vi "@create.vi"(4 "CodePage (<do not specify>)":i32(ring)=-1 items=["<do not specify>"=-1, "<use OEM Code Page>"=0, "IBM037 - IBM EBCDIC US-Canada"=37, "IBM437 - OEM United States"=437, "IBM500 - IBM EBCDIC International"=500, "ASMO-708 - Arabic (ASMO 708)"=708, "709 - Arabic (ASMO-449+, BCON V4)"=709, "710 - Arabic - Transparent Arabic"=710, "DOS-720 - Arabic (Transparent ASMO); Arabic (DOS)"=720, "ibm737 - OEM Greek (formerly 437G); Greek (DOS)"=737, "ibm775 - OEM Baltic; Baltic (DOS)"=775, "ibm850 - OEM Multilingual Latin 1; Western European (DOS)"=850, "ibm852 - OEM Latin 2; Central European (DOS)"=852, "IBM855 - OEM Cyrillic (primarily Russian)"=855, "ibm857 - OEM Turkish; Turkish (DOS)"=857, "IBM00858 - OEM Multilingual Latin 1 + Euro symbol"=858, "IBM860 - OEM Portuguese; Portuguese (DOS)"=860, "ibm861 - OEM Icelandic; Icelandic (DOS)"=861, "DOS-862 - OEM Hebrew; Hebrew (DOS)"=862, "IBM863 - OEM French Canadian; French Canadian (DOS)"=863, "IBM864 - OEM Arabic; Arabic (864)"=864, "IBM865 - OEM Nordic; Nordic (DOS)"=865, "cp866 - OEM Russian; Cyrillic (DOS)"=866, "ibm869 - OEM Modern Greek; Greek, Modern (DOS)"=869, "IBM870 - IBM EBCDIC Multilingual/ROECE (Latin 2); IBM EBCDIC Multilingual Latin 2"=870, "windows-874 - Thai (Windows)"=874, "cp875 - IBM EBCDIC Greek Modern"=875, "shift_jis - ANSI/OEM Japanese; Japanese (Shift-JIS)"=932, "gb2312 - ANSI/OEM Simplified Chinese (PRC, Singapore); Chinese Simplified (GB2312)"=936, "ks_c_5601-1987 - ANSI/OEM Korean (Unified Hangul Code)"=949, "big5 - ANSI/OEM Traditional Chinese (Taiwan; Hong Kong SAR, PRC); Chinese Traditional (Big5)"=950, "IBM1026 - IBM EBCDIC Turkish (Latin 5)"=1026, "IBM01047 - IBM EBCDIC Latin 1/Open System"=1047, "IBM01140 - IBM EBCDIC US-Canada (037 + Euro symbol); IBM EBCDIC (US-Canada-Euro)"=1140, "IBM01141 - IBM EBCDIC Germany (20273 + Euro symbol); IBM EBCDIC (Germany-Euro)"=1141, "IBM01142 - IBM EBCDIC Denmark-Norway (20277 + Euro symbol); IBM EBCDIC (Denmark-Norway-Euro)"=1142, "IBM01143 - IBM EBCDIC Finland-Sweden (20278 + Euro symbol); IBM EBCDIC (Finland-Sweden-Euro)"=1143, "IBM01144 - IBM EBCDIC Italy (20280 + Euro symbol); IBM EBCDIC (Italy-Euro)"=1144, "IBM01145 - IBM EBCDIC Latin America-Spain (20284 + Euro symbol); IBM EBCDIC (Spain-Euro)"=1145, "IBM01146 - IBM EBCDIC United Kingdom (20285 + Euro symbol); IBM EBCDIC (UK-Euro)"=1146, "IBM01147 - IBM EBCDIC France (20297 + Euro symbol); IBM EBCDIC (France-Euro)"=1147, "IBM01148 - IBM EBCDIC International (500 + Euro symbol); IBM EBCDIC (International-Euro)"=1148, "IBM01149 - IBM EBCDIC Icelandic (20871 + Euro symbol); IBM EBCDIC (Icelandic-Euro)"=1149, "utf-16 - Unicode UTF-16, little endian byte order (BMP of ISO 10646); available only to managed applications"=1200, "unicodeFFFE - Unicode UTF-16, big endian byte order; available only to managed applications"=1201, "windows-1250 - ANSI Central European; Central European (Windows)"=1250, "windows-1251 - ANSI Cyrillic; Cyrillic (Windows)"=1251, "windows-1252 - ANSI Latin 1; Western European (Windows)"=1252, "windows-1253 - ANSI Greek; Greek (Windows)"=1253, "windows-1254 - ANSI Turkish; Turkish (Windows)"=1254, "windows-1255 - ANSI Hebrew; Hebrew (Windows)"=1255, "windows-1256 - ANSI Arabic; Arabic (Windows)"=1256, "windows-1257 - ANSI Baltic; Baltic (Windows)"=1257, "windows-1258 - ANSI/OEM Vietnamese; Vietnamese (Windows)"=1258, "Johab - Korean (Johab)"=1361, "macintosh - MAC Roman; Western European (Mac)"=10000, "x-mac-japanese - Japanese (Mac)"=10001, "x-mac-chinesetrad - MAC Traditional Chinese (Big5); Chinese Traditional (Mac)"=10002, "x-mac-korean - Korean (Mac)"=10003, "x-mac-arabic - Arabic (Mac)"=10004, "x-mac-hebrew - Hebrew (Mac)"=10005, "x-mac-greek - Greek (Mac)"=10006, "x-mac-cyrillic - Cyrillic (Mac)"=10007, "x-mac-chinesesimp - MAC Simplified Chinese (GB 2312); Chinese Simplified (Mac)"=10008, "x-mac-romanian - Romanian (Mac)"=10010, "x-mac-ukrainian - Ukrainian (Mac)"=10017, "x-mac-thai - Thai (Mac)"=10021, "x-mac-ce - MAC Latin 2; Central European (Mac)"=10029, "x-mac-icelandic - Icelandic (Mac)"=10079, "x-mac-turkish - Turkish (Mac)"=10081, "x-mac-croatian - Croatian (Mac)"=10082, "utf-32 - Unicode UTF-32, little endian byte order; available only to managed applications"=12000, "utf-32BE - Unicode UTF-32, big endian byte order; available only to managed applications"=12001, "x-Chinese_CNS - CNS Taiwan; Chinese Traditional (CNS)"=20000, "x-cp20001 - TCA Taiwan"=20001, "x_Chinese-Eten - Eten Taiwan; Chinese Traditional (Eten)"=20002, "x-cp20003 - IBM5550 Taiwan"=20003, "x-cp20004 - TeleText Taiwan"=20004, "x-cp20005 - Wang Taiwan"=20005, "x-IA5 - IA5 (IRV International Alphabet No. 5, 7-bit); Western European (IA5)"=20105, "x-IA5-German - IA5 German (7-bit)"=20106, "x-IA5-Swedish - IA5 Swedish (7-bit)"=20107, "x-IA5-Norwegian - IA5 Norwegian (7-bit)"=20108, "us-ascii - US-ASCII (7-bit)"=20127, "x-cp20261 - T.61"=20261, "x-cp20269 - ISO 6937 Non-Spacing Accent"=20269, "IBM273 - IBM EBCDIC Germany"=20273, "IBM277 - IBM EBCDIC Denmark-Norway"=20277, "IBM278 - IBM EBCDIC Finland-Sweden"=20278, "IBM280 - IBM EBCDIC Italy"=20280, "IBM284 - IBM EBCDIC Latin America-Spain"=20284, "IBM285 - IBM EBCDIC United Kingdom"=20285, "IBM290 - IBM EBCDIC Japanese Katakana Extended"=20290, "IBM297 - IBM EBCDIC France"=20297, "IBM420 - IBM EBCDIC Arabic"=20420, "IBM423 - IBM EBCDIC Greek"=20423, "IBM424 - IBM EBCDIC Hebrew"=20424, "x-EBCDIC-KoreanExtended - IBM EBCDIC Korean Extended"=20833, "IBM-Thai - IBM EBCDIC Thai"=20838, "koi8-r - Russian (KOI8-R); Cyrillic (KOI8-R)"=20866, "IBM871 - IBM EBCDIC Icelandic"=20871, "IBM880 - IBM EBCDIC Cyrillic Russian"=20880, "IBM905 - IBM EBCDIC Turkish"=20905, "IBM00924 - IBM EBCDIC Latin 1/Open System (1047 + Euro symbol)"=20924, "EUC-JP - Japanese (JIS 0208-1990 and 0212-1990)"=20932, "x-cp20936 - Simplified Chinese (GB2312); Chinese Simplified (GB2312-80)"=20936, "x-cp20949 - Korean Wansung"=20949, "cp1025 - IBM EBCDIC Cyrillic Serbian-Bulgarian"=21025, "21027 - (deprecated)"=21027, "koi8-u - Ukrainian (KOI8-U); Cyrillic (KOI8-U)"=21866, "iso-8859-1 - ISO 8859-1 Latin 1; Western European (ISO)"=28591, "iso-8859-2 - ISO 8859-2 Central European; Central European (ISO)"=28592, "iso-8859-3 - ISO 8859-3 Latin 3"=28593, "iso-8859-4 - ISO 8859-4 Baltic"=28594, "iso-8859-5 - ISO 8859-5 Cyrillic"=28595, "iso-8859-6 - ISO 8859-6 Arabic"=28596, "iso-8859-7 - ISO 8859-7 Greek"=28597, "iso-8859-8 - ISO 8859-8 Hebrew; Hebrew (ISO-Visual)"=28598, "iso-8859-9 - ISO 8859-9 Turkish"=28599, "iso-8859-13 - ISO 8859-13 Estonian"=28603, "iso-8859-15 - ISO 8859-15 Latin 9"=28605, "x-Europa - Europa 3"=29001, "iso-8859-8-i - ISO 8859-8 Hebrew; Hebrew (ISO-Logical)"=38598, "iso-2022-jp - ISO 2022 Japanese with no halfwidth Katakana; Japanese (JIS)"=50220, "csISO2022JP - ISO 2022 Japanese with halfwidth Katakana; Japanese (JIS-Allow 1 byte Kana)"=50221, "iso-2022-jp - ISO 2022 Japanese JIS X 0201-1989; Japanese (JIS-Allow 1 byte Kana - SO/SI)"=50222, "iso-2022-kr - ISO 2022 Korean"=50225, "x-cp50227 - ISO 2022 Simplified Chinese; Chinese Simplified (ISO 2022)"=50227, "50229 - ISO 2022 Traditional Chinese"=50229, "50930 - EBCDIC Japanese (Katakana) Extended"=50930, "50931 - EBCDIC US-Canada and Japanese"=50931, "50933 - EBCDIC Korean Extended and Korean"=50933, "50935 - EBCDIC Simplified Chinese Extended and Simplified Chinese"=50935, "50936 - EBCDIC Simplified Chinese"=50936, "50937 - EBCDIC US-Canada and Traditional Chinese"=50937, "50939 - EBCDIC Japanese (Latin) Extended and Japanese"=50939, "euc-jp - EUC Japanese"=51932, "EUC-CN - EUC Simplified Chinese; Chinese Simplified (EUC)"=51936, "euc-kr - EUC Korean"=51949, "51950 - EUC Traditional Chinese"=51950, "hz-gb-2312 - HZ-GB2312 Simplified Chinese; Chinese Simplified (HZ)"=52936, "GB18030 - Windows XP and later: GB18030 Simplified Chinese (4 byte); Chinese Simplified (GB18030)"=54936, "x-iscii-de - ISCII Devanagari"=57002, "x-iscii-be - ISCII Bangla"=57003, "x-iscii-ta - ISCII Tamil"=57004, "x-iscii-te - ISCII Telugu"=57005, "x-iscii-as - ISCII Assamese"=57006, "x-iscii-or - ISCII Odia"=57007, "x-iscii-ka - ISCII Kannada"=57008, "x-iscii-ma - ISCII Malayalam"=57009, "x-iscii-gu - ISCII Gujarati"=57010, "x-iscii-pa - ISCII Punjabi"=57011, "utf-7 - Unicode (UTF-7)"=65000, "utf-8 - Unicode (UTF-8)"=65001], 6 "autorun? (false)":bool, 7 "dotnet_system_exec in":refnum<class "dotnet_system_exec.lvclass">, 8 "error in (no error)":errorcluster, 9 "working directory (c:\\)":path=path "c:/", 10 "arguments (\"\")":string, 11 "command line (cmd.exe)":string="cmd.exe") -> (0 "error out":errorcluster, 2 "public events":T1, 3 "dotnet_system_exec out":refnum<class "dotnet_system_exec.lvclass">)   [LabVIEW 2015, in "dotnet_system_exec.lvclass"]
doc: "Creates an instance of the .NET System Process. It configures the instance not to show a window but to redirect the stdout, stderr, and stdin so that LabVIEW can interface with them. Use the public events to register for the stdout and stderr events."
uses:
  dotnet_system_exec.lvclass
  dotnet_system_exec.lvclass/dotnet_system_exec.ctl
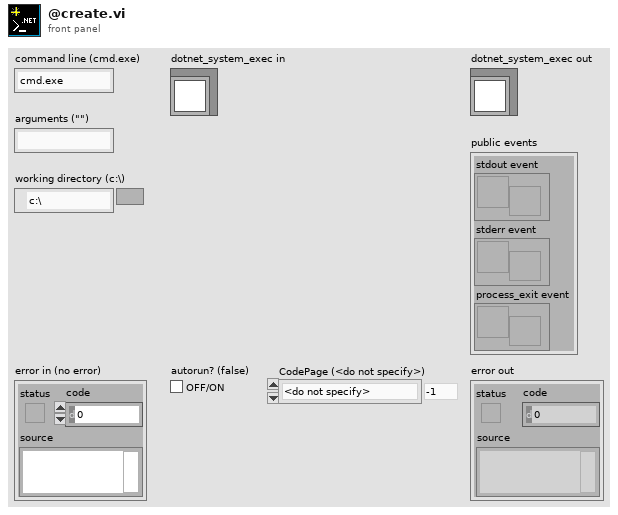
[diagram p1: front panel]
types:
  T1 = cluster{"stdout event":refnum<user-event>, "stderr event":refnum<user-event>, "process_exit event":refnum<user-event>}
  T2 = cluster{"StdOut Event":refnum<user-event>, "StdErr Event":refnum<user-event>, "ProcessExit Event":refnum<user-event>}
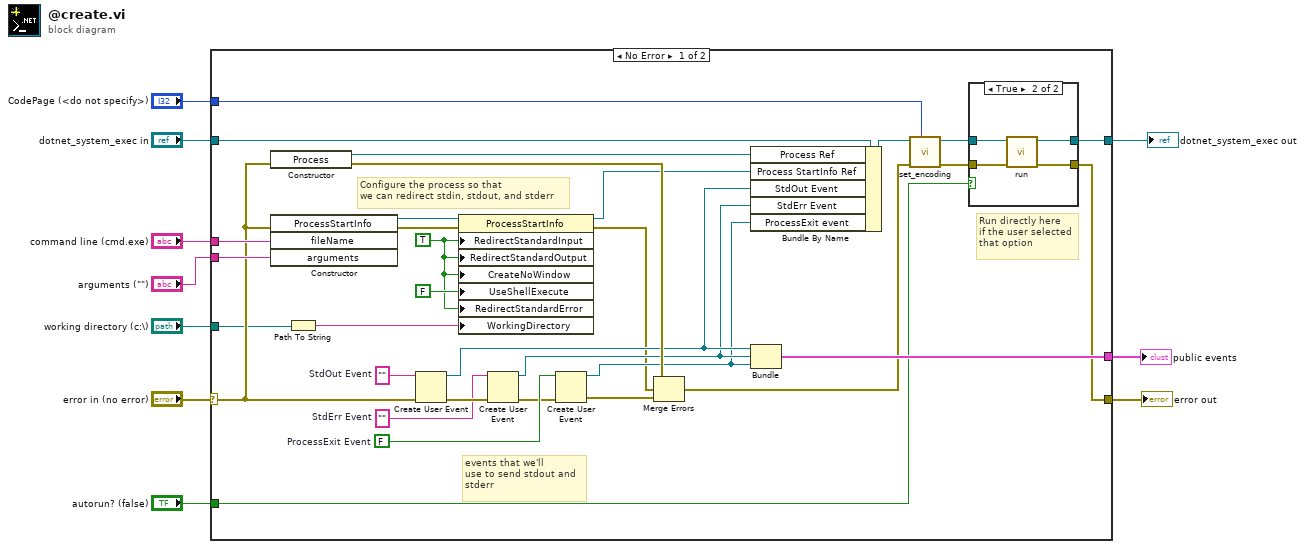
[diagram p0: block diagram]
diagram:
  n1 = case shown="No Error" "error in (no error)" {
    selector: "error in (no error)" -> [w29 w50]
    tunnel: [w23 w50] -> w9
    tunnel: [w24 w49] -> w7
    tunnel: "dotnet_system_exec in" -> [w34 w49]
    tunnel: "command line (cmd.exe)" -> [w37 _]
    tunnel: "arguments (\"\")" -> [w36 _]
    tunnel: "working directory (c:\\)" -> [w25 _]
    tunnel: [w28 _] -> w3
    tunnel: "autorun? (false)" -> [w22 _]
    tunnel: "CodePage (<do not specify>)" -> [w11 _]
    frame No Error {
      w21 = FALSE  # ProcessExit Event
      w30 = ""  # StdErr Event
      w32 = ""  # StdOut Event
      w39 = TRUE ("RedirectStandardInput")
      # "Configure the process so that\nwe can redirect stdin, stdout, and stderr"
      # "events that we'll\nuse to send stdout and\nstderr"
      # "Run directly here\nif the user selected\nthat option"
      n2 = constructor class="Process"(error in=w29) -> (reference out=w33:refnum<k24>, error out=w38:errorcluster)  [unwired: 2 in, 1 out]
      n3 = constructor class="ProcessStartInfo"(error in=w29, "fileName"=w37, "arguments"=w36) -> (reference out=w41:refnum<k24>, error out=w42:errorcluster)  [unwired: 2 in, 3 out]
      n4 = Path To String(path=w25) -> (string=w35:string)
      n5 = Create User Event(user event datatype=w32, error in=w29) -> (user event=w27:refnum<user-event>, error out=w31:errorcluster)
      n6 = property class="ProcessStartInfo"(reference=w41, error in=w42, "RedirectStandardInput"=w39, "RedirectStandardOutput"=w39, "CreateNoWindow"=w39, "UseShellExecute"=FALSE, "RedirectStandardError"=w39, "WorkingDirectory"=w35) -> (reference out=w17:refnum<k24>, error out=w16:errorcluster)
      n7 = Create User Event(user event datatype=w30, error in=w31) -> (user event=w26:refnum<user-event>, error out=w20:errorcluster)
      n8 = Create User Event(user event datatype=w21, error in=w20) -> (user event=w18:refnum<user-event>, error out=w19:errorcluster)
      n9 = Merge Errors(w38, w16, w19) -> (w15:errorcluster)
      n10 = Bundle By Name(cluster=w34, "Process Ref"=w33, "Process StartInfo Ref"=w17, "StdOut Event"=w27, "StdErr Event"=w26, "ProcessExit event"=w18) -> (w13:refnum<class "dotnet_system_exec.lvclass">)
      n11 = Bundle("StdOut Event"=w27, "StdErr Event"=w26, "ProcessExit Event"=w18) -> (w28:T2)  [unwired: 1 in]
      n12 = call "set_encoding.vi"("CodePage"=w11, "error in (no error)"=w15, "dotnet_system_exec.lvclass in"=w13) -> ("error out"=w14:errorcluster, "dotnet_system_exec.lvclass out"=w12:refnum<class "dotnet_system_exec.lvclass">)  [unwired: 7 in]
      n13 = case shown="True" w22 {
        tunnel: w12 -> [w44 w48]
        tunnel: [w44 w47] -> w24
        tunnel: w14 -> [w43 w46]
        tunnel: [w43 w45] -> w23
        frame False {
        }
        frame True {
          n14 = call "run.vi"("error in (no error)"=w46, "dotnet_system_exec in"=w48) -> ("error out"=w45:errorcluster, "dotnet_system_exec out"=w47:refnum<class "dotnet_system_exec.lvclass">)  [unwired: 8 in]
        }
      }
    }
    frame Error {
    }
  }
  "error out" <- w9
  "dotnet_system_exec out" <- w7
  "public events" <- w3
